vi "thcd_set_gid.vi"(5 "thcd_delay":u32=500, 6 "err_in":errorcluster, 7 "thcd_val":T1, 8 "thcd_ch":T2, 9 "thcd_visa":refnum<visa-resource-name>) -> (0 "err_out":errorcluster, 1 "thcd_st":bool, 2 "thcd_res_msg":string, 3 "thcd_visa":refnum<visa-resource-name>)   [LabVIEW 2020, in "1039_mod.lvlib"]
uses:
  1039_mod/1039_mod.lvlib
  thcd_controls/ctrl_chn_thcd.ctl
  thcd_controls/ctrl_gid_thcd.ctl
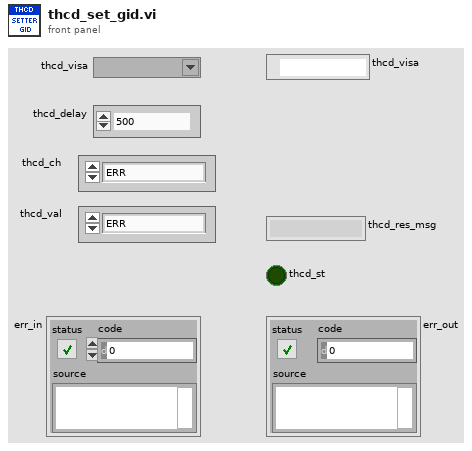
[diagram p1: front panel]
types:
  T1 = typedef "ctrl_gid_thcd.ctl" = enum16{"ERR", "1", "2", "C3H6O_1", "C2H3N", "C2H2", "Air", "C3H4_1", "NH3", "Ar", "AsH3", "C6H6", "BCl3", "BF3", "Br2", "15", "16", "CBrF3", "C4H10_1", "19", "C4H8_1", "CO2", "CS2", "CO", "CCl4", "COS", "Cl2", "ClF3", "28", "29", "CHCl3", "31", "32", "C4H8_2", "C2N2", "ClCN", "C4H8_3", "C3H6", "H22", "B2H6", "40", "R21", "42", "43", "44", "45", "46", "47", "48", "C2H7N_1", "C2H6O_1", "C2H6S_1", "C4H6_1", "C2H6", "54", "55", "C2H6O_2", "C4H6_2", "C2H7N_2", "C8H10", "60", "61", "C2H5F", "C2H4", "64", "65", "C2H4O", "C2H4N", "68", "C2H6S_2", "F2", "CH2O", "CCl3F", "73", "CClF3", "CF4", "76", "CHF3", "78", "C4H4O", "He", "C3HF7", "HMDS", "83", "C6H14", "C6F6", "C6H12_1", "N2H4", "H2", "HBr", "HCl", "CHN", "HF", "HI", "H2Se", "H2S", "C4H10_2", "97", "C4H8_4", "C5H12_1", "C3H8O_1", "101", "C2H2O", "Kr", "CH4", "CH4O", "106", "C3H4_2", "CH5N", "CH3Br", "CH3Cl", "C7H14", "C3H9N", "C3H8O_2", "C3H8S", "CH3F", "116", "CH3I", "CH4S", "C6H12_2", "C3H6O_2", "Ne", "NO", "N2", "NO2", "N2O4", "NF3", "127", "NOCl", "N2O", "C5H12_2", "C8H18", "O2", "F2O", "O3", "B5H9", ""}
  T2 = typedef "ctrl_chn_thcd.ctl" = enum8{"ERR", "1", "2", "3", "4"}
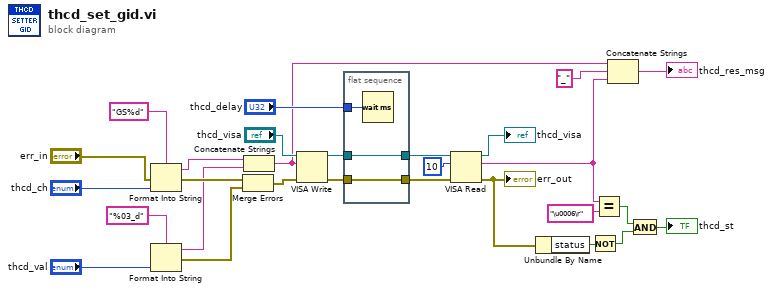
[diagram p0: block diagram]
diagram:
  n1 = Format Into String(format string="GS%d", error in="err_in", "thcd_ch") -> (resulting string=w20:string, error out=w19:errorcluster)  [unwired: 1 in]
  n2 = Format Into String(format string="%03_d", "thcd_val") -> (resulting string=w16:string, error out=w17:errorcluster)  [unwired: 2 in]
  n3 = Merge Errors(w19, w17) -> (w18:errorcluster)
  n4 = Concatenate Strings(w20, w16) -> (w3:string)
  n5 = VISA Write(VISA resource name="thcd_visa", write buffer=w3, error in (no error)=w18) -> (VISA resource name out=w27:refnum<visa-resource-name>, error out=w28:errorcluster)  [unwired: 1 out]
  n6 = flat-sequence {
    tunnel: w28 -> [w30]
    tunnel: [w30] -> w6
    tunnel: w27 -> [w29]
    tunnel: [w29] -> w7
    tunnel: "thcd_delay" -> [w31]
    frame #0 {
      n7 = Wait (ms)(milliseconds to wait=w31) -> ()  [unwired: 1 out]
    }
  }
  n8 = VISA Read(VISA resource name=w7, byte count=u32 10, error in (no error)=w6) -> (VISA resource name out=→"thcd_visa":refnum<visa-resource-name>, read buffer=w8:string, error out=w4:errorcluster)  [unwired: 1 out]
  "err_out" <- w4
  n9 = Unbundle By Name(w4) -> ("status"=w14:bool)
  n10 = Not(x=w14) -> (.not. x?=w11:bool)
  n11 = Equal?(x=w8, y="\u0006\r") -> (x = y?=w12:bool)
  n12 = Concatenate Strings(w3, "_", w8) -> (→"thcd_res_msg":string)
  n13 = And(x=w12, y=w11) -> (x .and. y?=→"thcd_st":bool)
